vi "Read Measurements.vi"(8 "error in (no error)":errorcluster, 11 "Abs Instrument in":refnum<class "Power Supply Instrument.lvclass">) -> (0 "error out":errorcluster, 2 "Measurements":T1[](array[typedef]) {"Lower limit" format="%#_4p"; "Upper limit" format="%#_4p"}, 3 "Abs Instrument out":refnum<class "Power Supply Instrument.lvclass">)   [LabVIEW 2025, in "Power Supply.lvlib" / "Power Supply Instrument.lvclass"]
uses:
  Power Supply Instrument.lvclass
  Power Supply Instrument.lvclass/Power Supply Instrument.ctl
  <vilib>/Analysis/NI_AALBase.lvlib
  <vilib>/Analysis/baseanly.llb/Mean (DBL).vi
  Users/Public/Documents/Sandia National Labs/TSS Plugin/Abstract Engine.lvlibp/Abstract Instrument/Channel.ctl
  Users/Public/Documents/Sandia National Labs/TSS Plugin/Abstract Engine.lvlibp/Abstract Instrument/Abstract Instrument.lvclass
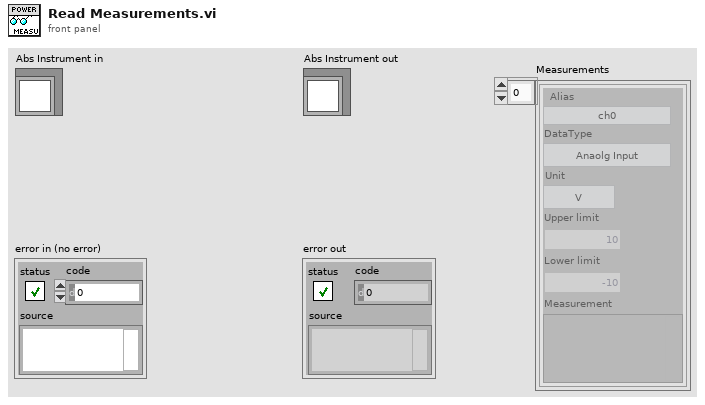
[diagram p1: front panel]
types:
  T1 = typedef "Abstract Engine.lvlibp/Abstract Instrument.lvclass/Channel.ctl" = cluster{"Alias":string, "DataType":enum16{"Anaolg Input", "Waveform"}, "Unit":enum16{"---", "V", "A", "Ohm", "Hz", "uF", "degC", "deg"}, "Upper limit":dbl, "Lower limit":dbl, "Measurement":variant}
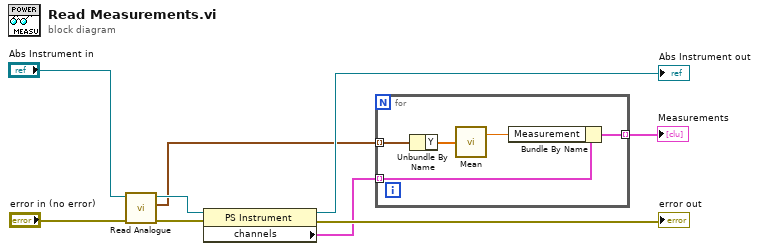
[diagram p0: block diagram]
diagram:
  n1 = call-dynamic "Read Analogue.vi"("error in (no error)"="error in (no error)", "PS Instrument"="Abs Instrument in") -> ("error out"=w7:errorcluster, "Waveforms"=w1:waveform(dbl)[], "PS Instrument out"=w6:refnum<class "Power Supply Instrument.lvclass">)  [unwired: 7 in]
  n2 = property class="PS Instrument"(reference=w6, error in=w7) -> (reference out=→"Abs Instrument out":refnum<class "Power Supply Instrument.lvclass">, error out=→"error out":errorcluster, "channels"=w3:T1[])
  n3 = for {
    tunnel: w3 -> [w13] mode=indexing
    tunnel: [w14] -> w2 mode=indexing
    tunnel: w1 -> [w12] mode=indexing
    n4 = Unbundle By Name(w12) -> ("Y"=w11:dbl[])
    n5 = call-poly <vilib>:"Mean.vi"("X"=w11) -> ("mean"=w10:dbl)  [unwired: 1 out]
    n6 = Bundle By Name(cluster=w13, "Measurement"=w10) -> (w14:T1)
  }
  "Measurements" <- w2
